vi "Clear Selections.vi"(8 "error in (no error)":errorcluster, 11 "FSM in":refnum<class "FSM.Graph.lvclass">) -> (0 "error out":errorcluster, 3 "FSM out":refnum<class "FSM.Graph.lvclass">)   [LabVIEW 2015, in "FSM.Graph.lvclass"]
uses:
  FSM.Graph.lvclass
  FSM.Graph.lvclass/FSM.Graph.ctl
  FSM.Node/FSM.Node.lvclass/FSM.Node.ctl
  FSM.Node/Write selected.vi
  FSM.Node/FSM.Node.lvclass
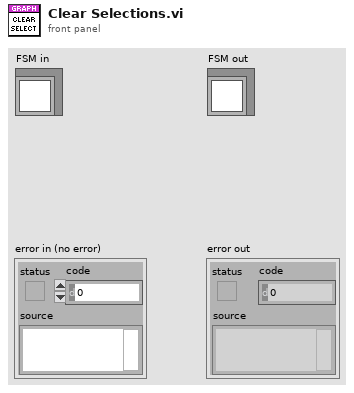
[diagram p1: front panel]
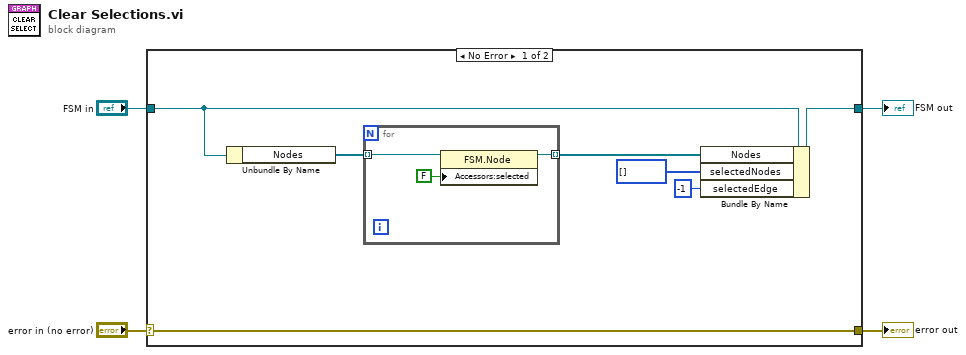
[diagram p0: block diagram]
diagram:
  n1 = case shown="No Error" "error in (no error)" {
    selector: "error in (no error)" -> [w11 w16]
    tunnel: [w11 w16] -> w3
    tunnel: [w8 w15] -> w1
    tunnel: "FSM in" -> [w10 w15]
    frame No Error {
      n2 = Unbundle By Name(w10) -> ("Nodes"=w9:refnum<class "FSM.Node.lvclass">[])
      n3 = for {
        tunnel: w9 -> [w14] mode=indexing
        tunnel: [w13] -> w7 mode=indexing
        n4 = property class="FSM.Node"(reference=w14, "Accessors:selected"=FALSE ("selected")) -> (reference out=w13:refnum<class "FSM.Node.lvclass">)  [unwired: 1 in, 1 out]
      }
      n5 = Bundle By Name(cluster=w10, "Nodes"=w7, "selectedNodes"=i32[] [], "selectedEdge"=-1) -> (w8:refnum<class "FSM.Graph.lvclass">)
    }
    frame Error {
    }
  }
  "error out" <- w3
  "FSM out" <- w1
